vi "(SubVI) Pairwise.vi"(4 "Data":dbl[](array[numeric])) -> (1 "Pairwise":dbl[](array[numeric]))   [LabVIEW 2014]
uses:
  <vilib>/Analysis/NI_AALBase.lvlib
panel:
  out "Histogram Graph":T1(graph)
  out "Waveform Graph":dbl[](graph)
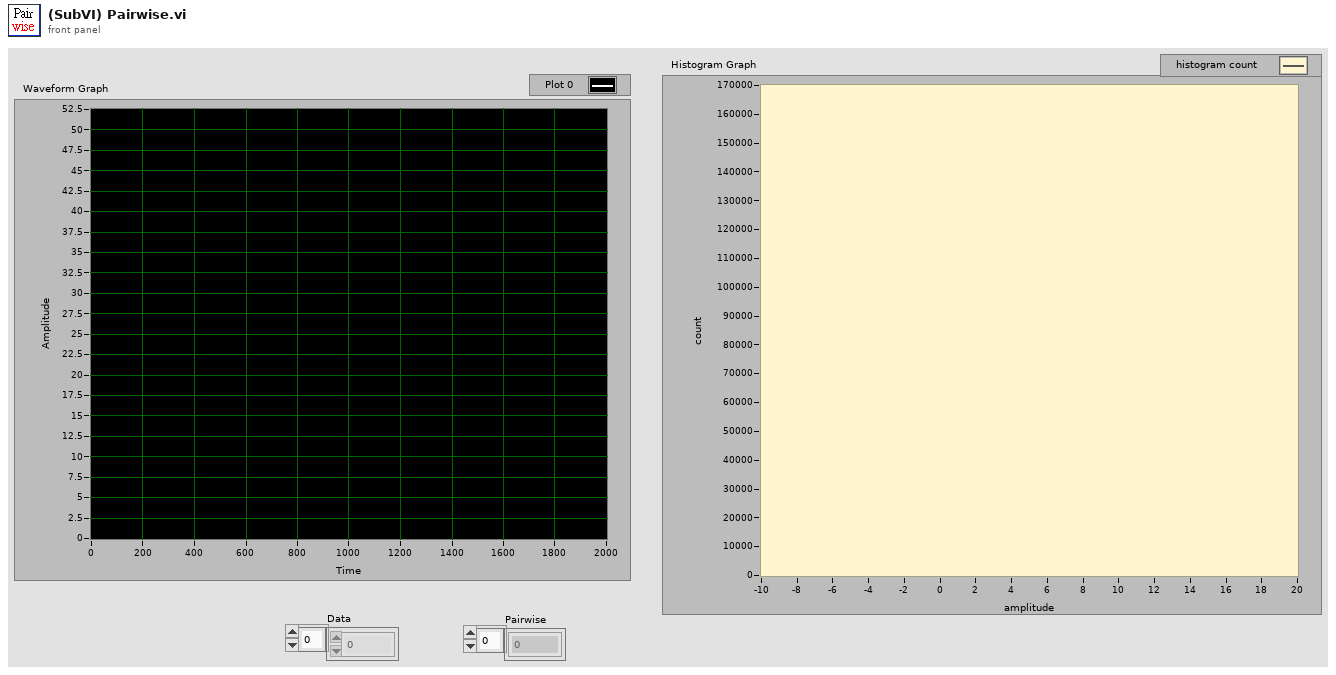
[diagram p1: front panel]
types:
  T1 = cluster{"X Values":dbl[], "Histogram: h(x)":i32[]}
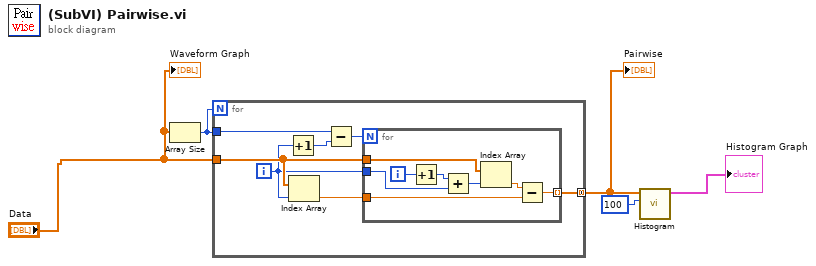
[diagram p0: block diagram]
diagram:
  n1 = Array Size(array="Data") -> (size(s)=w5:i32)
  n2 = for {
    N: w5 -> [_]
    tunnel: "Data" -> [w10]
    tunnel: [w11] -> w4 mode=concatenating
    tunnel: w5 -> [w8]
    i -> [w6]
    n3 = Increment(x=w6) -> (x+1=w7:i32)
    n4 = Index Array(array=w10, index=w6) -> (element=w12:dbl)
    n5 = Subtract(x=w8, y=w7) -> (x-y=w9:i32)
    n6 = for {
      N: w9 -> [_]
      tunnel: w12 -> [w17]
      tunnel: w10 -> [w20]
      tunnel: [w16] -> w11 mode=indexing
      tunnel: w6 -> [w14]
      i -> [w19]
      n7 = Increment(x=w19) -> (x+1=w15:i32)
      n8 = Add(x=w15, y=w14) -> (x+y=w13:i32)
      n9 = Index Array(array=w20, index=w13) -> (element=w18:dbl)
      n10 = Subtract(x=w18, y=w17) -> (x-y=w16:dbl)
    }
  }
  "Pairwise" <- w4
  n11 = call <vilib>:"Histogram.vi"("intervals"=100, "X"=w4) -> ("Histogram Graph"=→"Histogram Graph":T1)  [unwired: 6 in, 3 out]
  "Waveform Graph" <- "Data"
